vi "main.vi"() -> ()   [LabVIEW 2023]
uses:
  <vilib>/Analysis/2dsp.llb/1D Convolution (DBL).vi
  <vilib>/Analysis/NI_AALPro.lvlib
panel:
  out "Exponential window (using convolution)":dbl[][](graph)
  in  "a":dbl=0.4 min=0.0 max=1.0
  out "Square window (using convolution)":dbl[][](graph)
  out "Array 2":dbl[](array[numeric])
  out "Square window (my realization)":dbl[][](graph)
  out "Array":dbl[](array[numeric])
  in  "L":u16=20 step=1
  out "Input Array":dbl[](array[numeric])
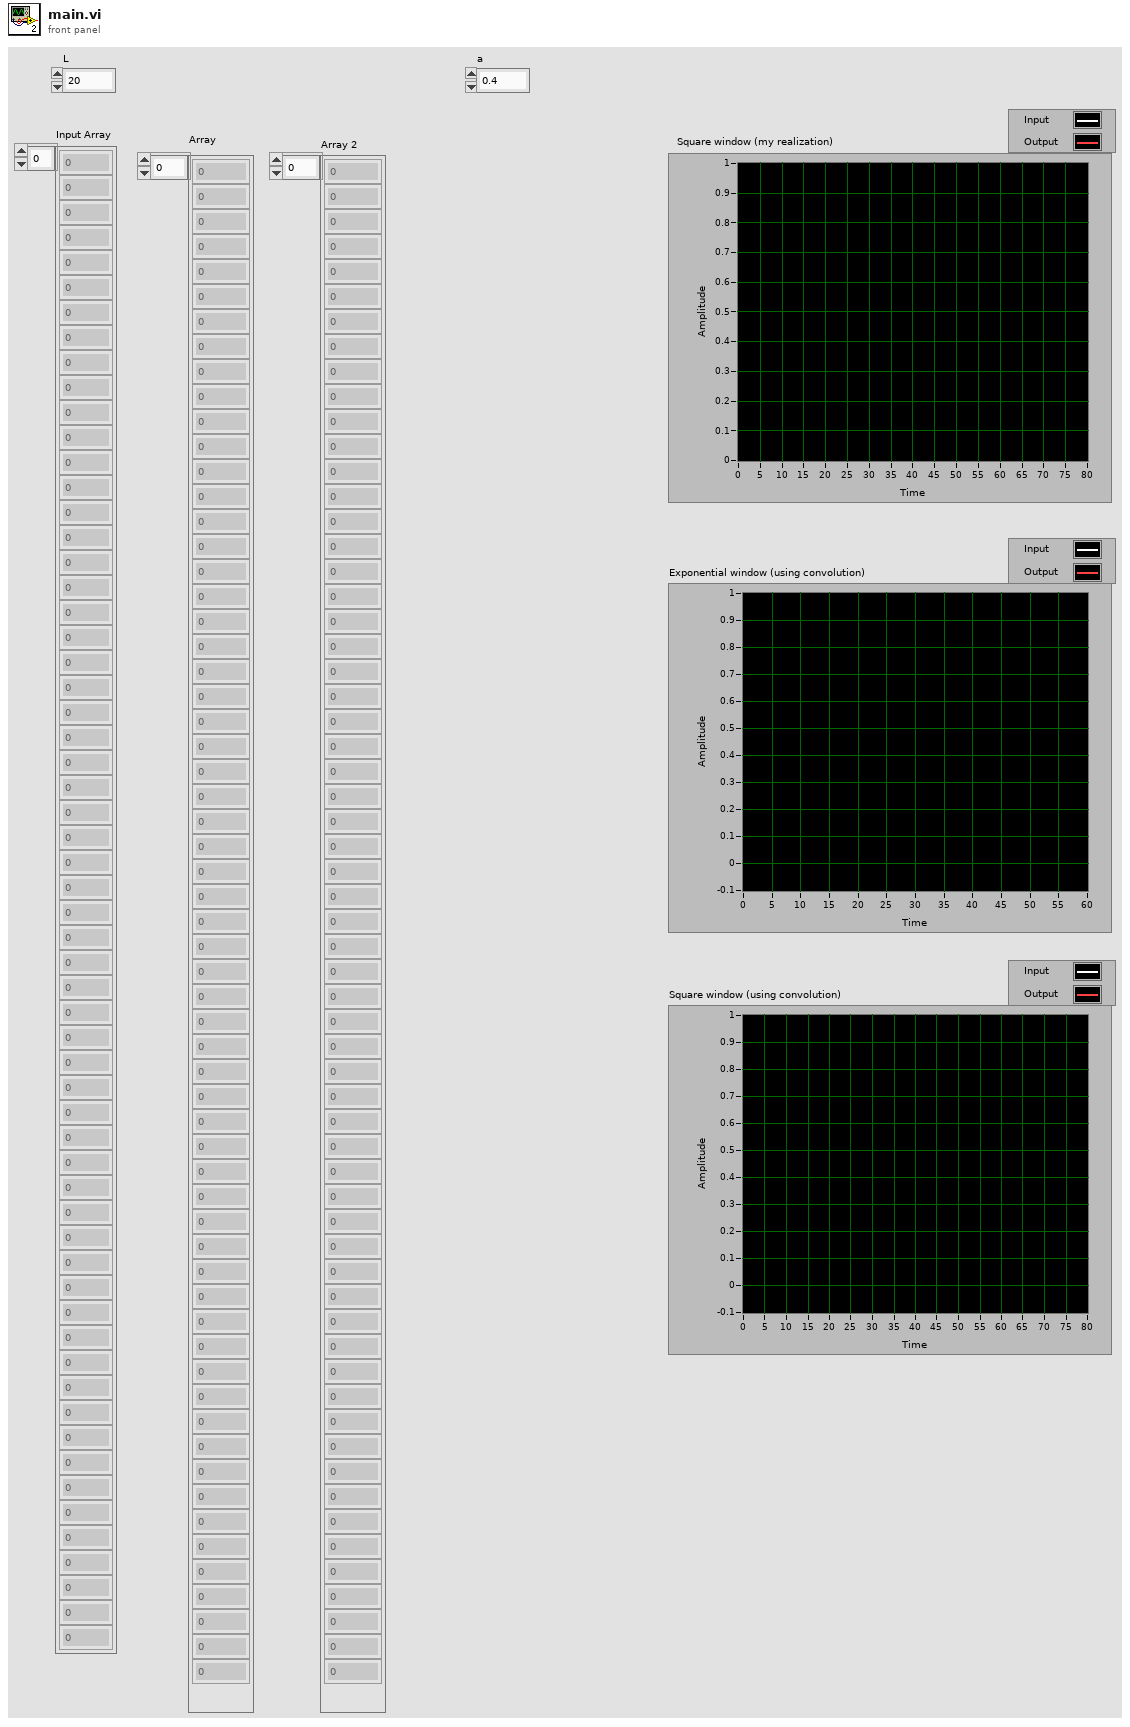
[diagram p1: front panel]
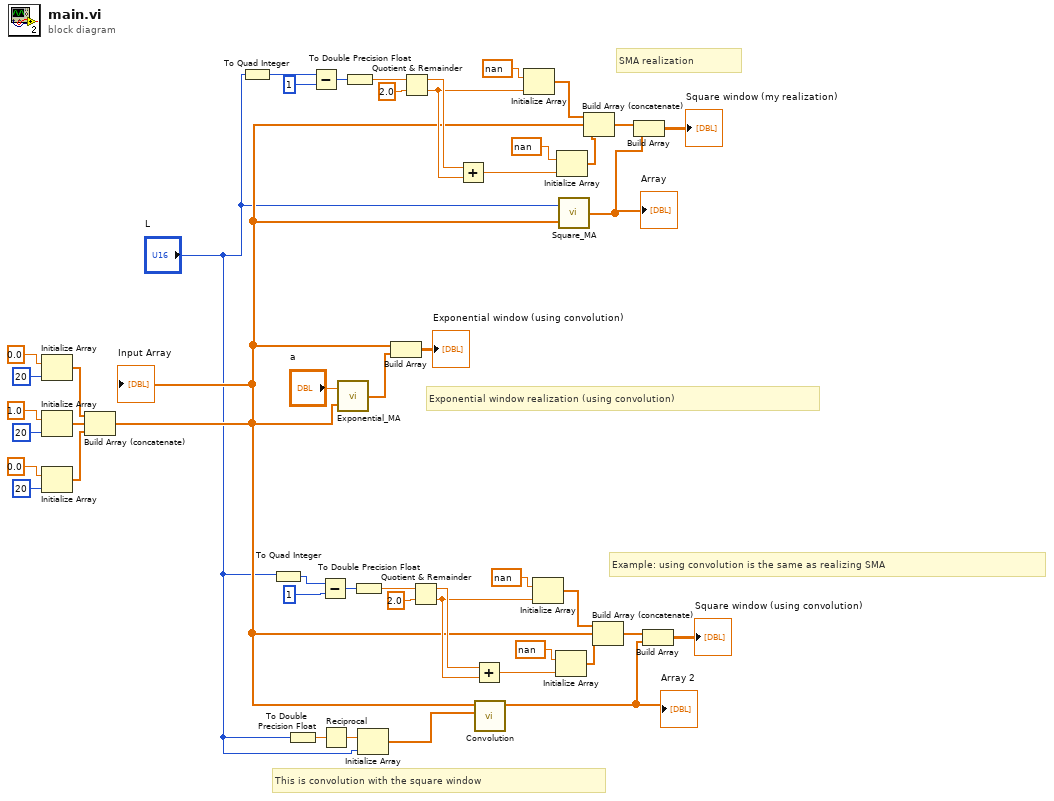
[diagram p0: block diagram]
diagram:
  # "This is convolution with the square window"
  # "SMA realization"
  # "Exponential window realization (using convolution)"
  # "Example: using convolution is the same as realizing SMA"
  n1 = Initialize Array(0.0 ("element"), 20 ("dimension size")) -> (w41:dbl[])
  n2 = Initialize Array(1.0 ("element"), 20 ("dimension size")) -> (w40:dbl[])
  n3 = Initialize Array(0.0 ("element"), 20 ("dimension size")) -> (w39:dbl[])
  n4 = Build Array (concatenate)(w41, w40, w39) -> (w3:dbl[])
  "Input Array" <- w3
  n5 = To Quad Integer(1:"L") -> (0:w35:i64)
  n6 = To Quad Integer(1:"L") -> (0:w2:i64)
  n7 = To Double Precision Float(number="L") -> (double precision float=w22:dbl)
  n8 = Subtract(x=w35, y=i64 1) -> (x-y=w36:i64)
  n9 = Subtract(x=w2, y=i64 1) -> (x-y=w18:i64)
  n10 = Reciprocal(x=w22) -> (1/x=w23:dbl)
  n11 = call "Exponential_MA.vi"("Input Array"=w3, "a"="a") -> ("Output Array"=w4:dbl[])
  n12 = To Double Precision Float(number=w36) -> (double precision float=w32:dbl)
  n13 = To Double Precision Float(number=w18) -> (double precision float=w15:dbl)
  n14 = Initialize Array(w23, "L") -> (w21:dbl[])
  n15 = Build Array(w3, w4) -> (→"Exponential window (using convolution)":dbl[][])
  n16 = Quotient & Remainder(x=w32, y=2.0) -> (x-y*floor(x/y)=w28:dbl, floor(x/y)=w27:dbl)
  n17 = Quotient & Remainder(x=w15, y=2.0) -> (x-y*floor(x/y)=w11:dbl, floor(x/y)=w10:dbl)
  n18 = Add(x=w28, y=w27) -> (x+y=w26:dbl)
  n19 = Add(x=w11, y=w10) -> (x+y=w9:dbl)
  n20 = call-poly <vilib>:"Convolution.vi"("Y"=w21, "X"=w3) -> ("X * Y"=w7:dbl[])  [unwired: 8 in, 1 out]
  "Array 2" <- w7
  n21 = Initialize Array(nan, w27) -> (w33:dbl[])
  n22 = Initialize Array(nan, w10) -> (w16:dbl[])
  n23 = Initialize Array(nan, w9) -> (w12:dbl[])
  n24 = Initialize Array(nan, w26) -> (w29:dbl[])
  n25 = call "Square_MA.vi"("Input Array"=w3, "L"="L") -> ("Output Array"=w24:dbl[])
  "Array" <- w24
  n26 = Build Array (concatenate)(w33, w3, w29) -> (w30:dbl[])
  n27 = Build Array (concatenate)(w16, w3, w12) -> (w13:dbl[])
  n28 = Build Array(w30, w24) -> (→"Square window (my realization)":dbl[][])
  n29 = Build Array(w13, w7) -> (→"Square window (using convolution)":dbl[][])
